vi "appendXMLName.vi"(7 "error in (no error)":errorcluster, 9 "name":string, 10 "Parent Device Node":refnum<k20>, 11 "DOM document in":refnum<k20>) -> (0 "error out":errorcluster)   [LabVIEW 2013]
uses:
  <resource>/objmgr/DOMUserDefRef.rc
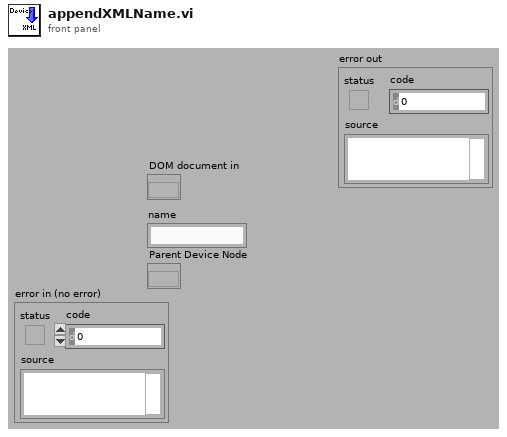
[diagram p1: front panel]
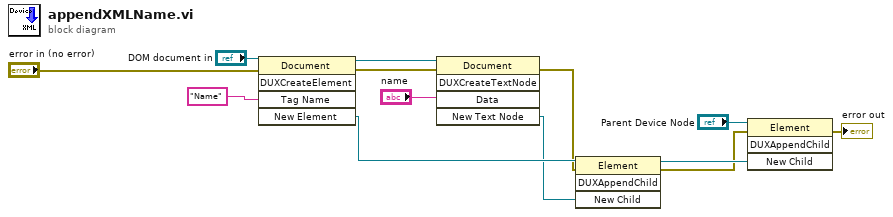
[diagram p0: block diagram]
diagram:
  n1 = invoke class="Document" method="DUXCreateElement"(reference="DOM document in", error in="error in (no error)", "Tag Name"="Name") -> (reference out=w12:refnum<k20>, error out=w4:errorcluster, "New Element"=w9:refnum<k20>)  [unwired: 2 in, 2 out]
  n2 = invoke class="Document" method="DUXCreateTextNode"(reference=w12, error in=w4, "Data"="name") -> (error out=w3:errorcluster, "New Text Node"=w8:refnum<k20>)  [unwired: 2 in, 3 out]
  n3 = invoke class="Element" method="DUXAppendChild"(reference=w9, error in=w3, "New Child"=w8) -> (reference out=w6:refnum<k20>, error out=w2:errorcluster)  [unwired: 1 in, 2 out]
  n4 = invoke class="Element" method="DUXAppendChild"(reference="Parent Device Node", error in=w2, "New Child"=w6) -> (error out=→"error out":errorcluster)  [unwired: 1 in, 3 out]
